vi "TEST_plot_table.vi"() -> ()   [LabVIEW 2025]
panel:
  in  "Table Control":string[][](table)
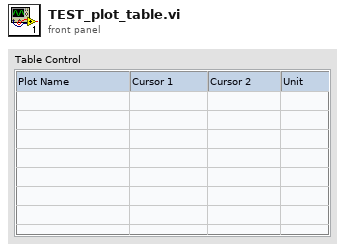
[diagram p1: front panel]
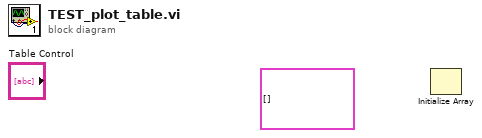
[diagram p0: block diagram]
diagram:
  (unwired) cluster{"Y":dbl[], "X2":dbl[]}[] [] ("graph_data")
  n1 = Initialize Array() -> ()  [unwired: 2 in, 1 out]
